vi "Nahid Final.vi"() -> ()   [LabVIEW 2019]
uses:
  <vilib>/robotics/Controls/Attitude Indicator/Attitude Indicator.xctl
  <vilib>/robotics/Controls/Compass Indicator/Compass Indicator.xctl
  <vilib>/Instr/_visa.llb/VISA Configure Serial Port (Instr).vi
panel:
  in  "byte count":u32
  in  "Speed":u32
  in  "VISA resource name":refnum<visa-resource-name>
  out "read buffer":string
  in  "Stop Button":bool
  out "Accelerometer Z":dynamicdata(graph)
  out "Accelerometer Y":dynamicdata(graph)
  out "Accelerometer X":dynamicdata(graph)
  out "Gyroscope Z":dynamicdata(graph)
  out "Gyroscope Y":dynamicdata(graph)
  out "Gyroscope X":dynamicdata(graph)
  out "Direction":dbl
  out "Thermometer":dbl(slide) scale=-2.0..100.0
  out "Low":bool
  out "Moderate":bool
  out "High":bool
  out "Temperature":dbl
  out "Humidity":dbl(slide) scale=0.0..100.0
  out "Yaw":dbl
  out "Pitch":dbl
  out "Roll":dbl
  out "Acc  Z":dbl
  out "Acc  Y":dbl
  out "Acc  X":dbl
  out "Gyro Z":dbl
  out "Gyro Y":dbl
  out "Gyro X":dbl
  out "Pressure":dbl(knob) scale=0.0..100.0
  out "Pressure":dbl
  out "Humidity":dbl
  out "Compass Indicator":dbl(xcontrol)
  out "Attitude Indicator":cluster{"Roll":dbl, "Pitch":dbl}(xcontrol)
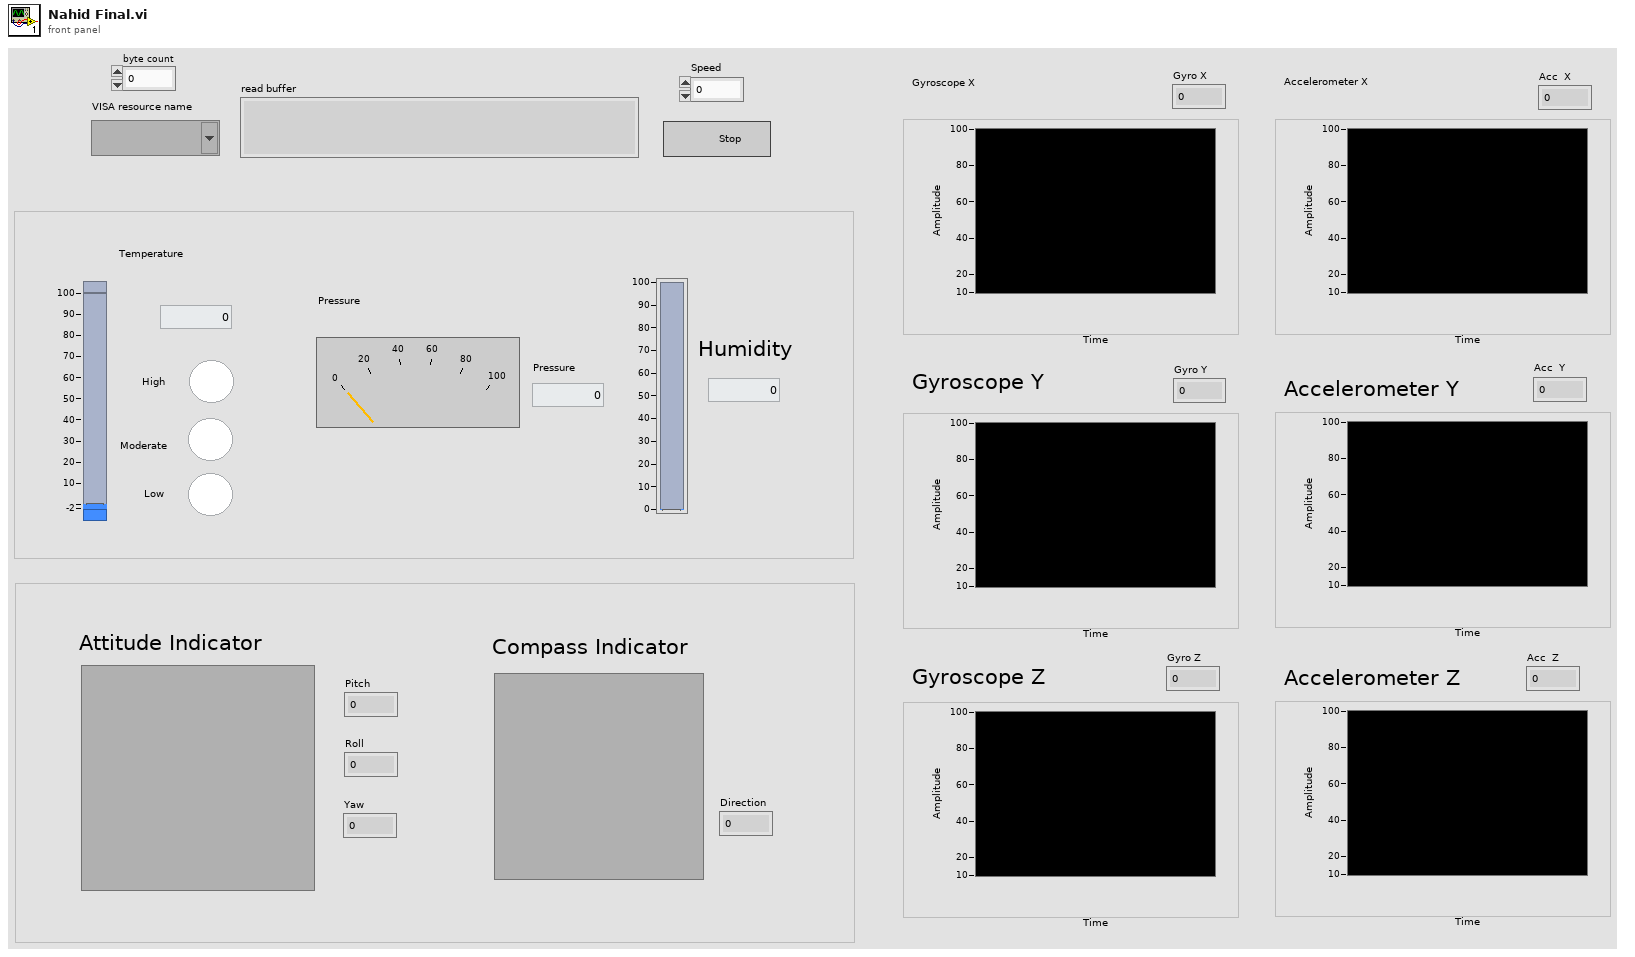
[diagram p1: front panel]
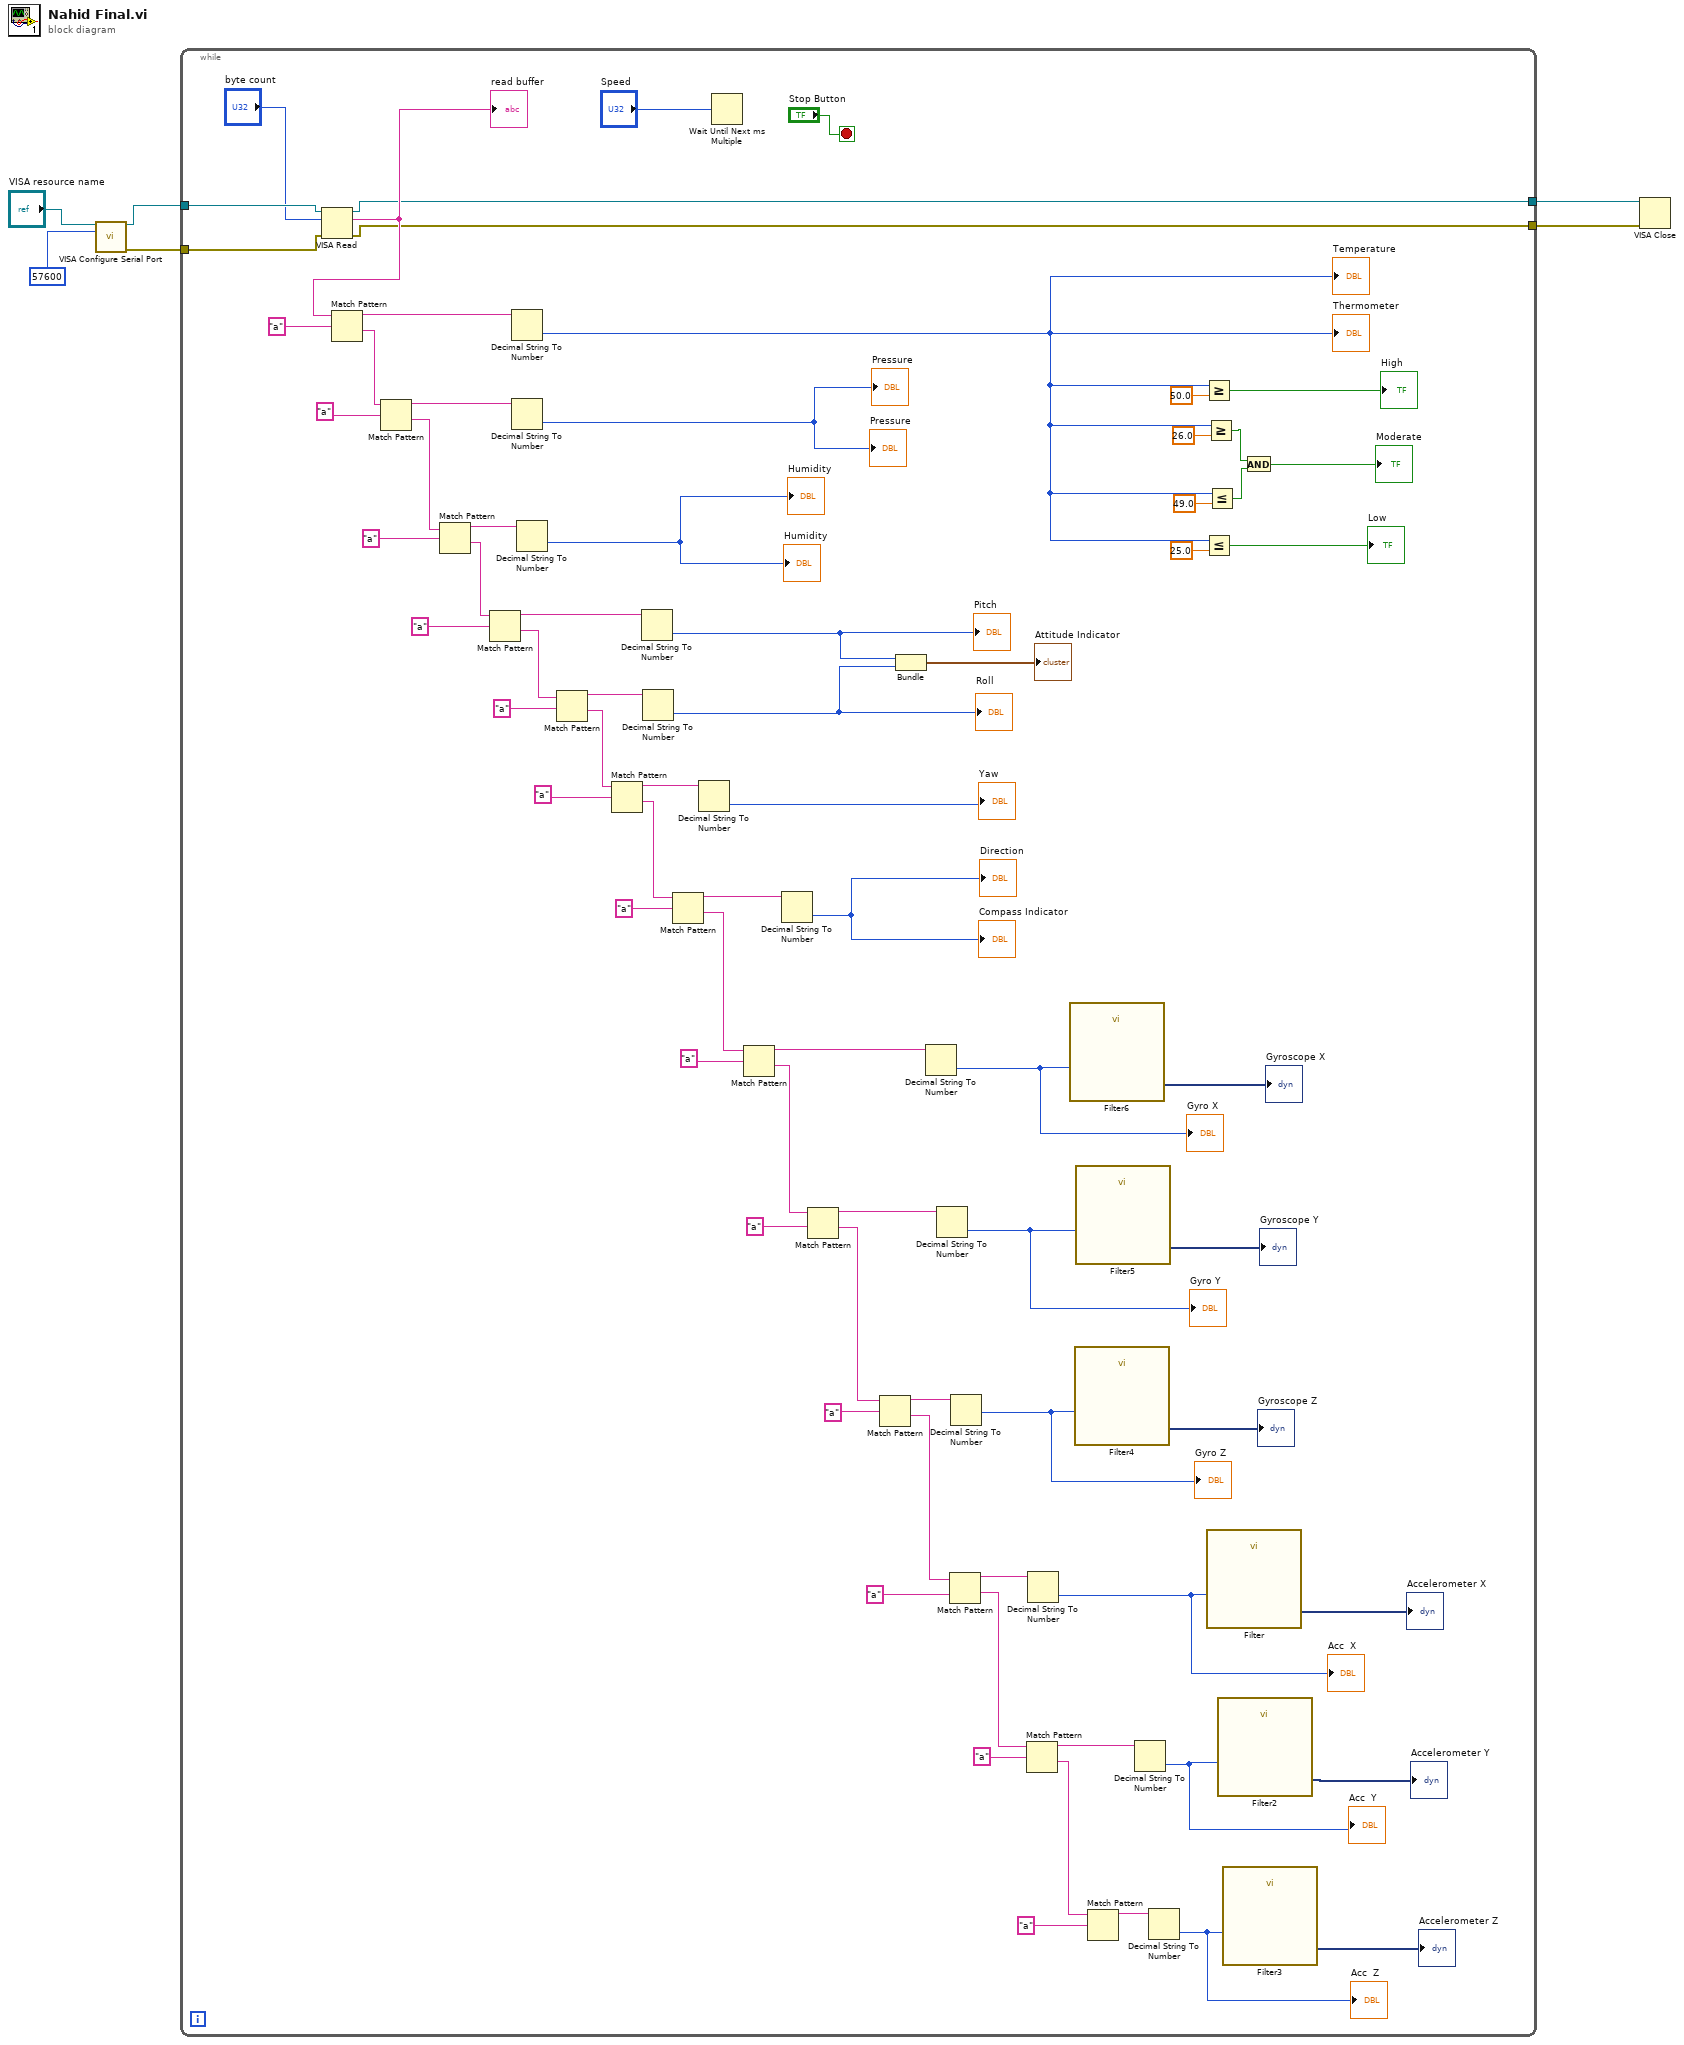
[diagram p0: block diagram]
diagram:
  n1 = call-poly "VISA Configure Serial Port"("VISA resource name"="VISA resource name", "baud rate (9600)"=u32 57600) -> ("VISA resource name out"=w4:refnum<visa-resource-name>, "error out"=w3:errorcluster)  [unwired: 12 in]
  n2 = while {
    tunnel: w4 -> [w63]
    tunnel: w3 -> [w62]
    tunnel: [w61] -> w2
    tunnel: [w60] -> w1
    stop <- "Stop Button" stop-if-true
    n3 = VISA Read(VISA resource name=w63, byte count="byte count", error in (no error)=w62) -> (VISA resource name out=w61:refnum<visa-resource-name>, read buffer=w68:string, error out=w60:errorcluster)  [unwired: 1 out]
    "read buffer" <- w68
    n4 = Match Pattern(string=w68, regular expression="a") -> (before substring=w65:string, after substring=w18:string)  [unwired: 1 in, 2 out]
    n5 = Match Pattern(string=w18, regular expression="a") -> (before substring=w70:string, after substring=w66:string)  [unwired: 1 in, 2 out]
    n6 = Match Pattern(string=w66, regular expression="a") -> (before substring=w64:string, after substring=w67:string)  [unwired: 1 in, 2 out]
    n7 = Match Pattern(string=w67, regular expression="a") -> (before substring=w58:string, after substring=w53:string)  [unwired: 1 in, 2 out]
    n8 = Decimal String To Number(string=w65) -> (number=w59:i32)  [unwired: 2 in, 1 out]
    "Temperature" <- w59
    "Thermometer" <- w59
    n9 = Decimal String To Number(string=w70) -> (number=→"Pressure" →"Pressure":i32)  [unwired: 2 in, 1 out]
    n10 = Decimal String To Number(string=w64) -> (number=→"Humidity" →"Humidity":i32)  [unwired: 2 in, 1 out]
    n11 = Match Pattern(string=w53, regular expression="a") -> (before substring=w56:string, after substring=w57:string)  [unwired: 1 in, 2 out]
    n12 = Match Pattern(string=w57, regular expression="a") -> (before substring=w54:string, after substring=w38:string)  [unwired: 1 in, 2 out]
    n13 = Decimal String To Number(string=w58) -> (number=w8:i32)  [unwired: 2 in, 1 out]
    "Pitch" <- w8
    n14 = Decimal String To Number(string=w56) -> (number=w52:i32)  [unwired: 2 in, 1 out]
    "Roll" <- w52
    n15 = Match Pattern(string=w38, regular expression="a") -> (before substring=w46:string, after substring=w49:string)  [unwired: 1 in, 2 out]
    n16 = Decimal String To Number(string=w54) -> (number=→"Yaw":i32)  [unwired: 2 in, 1 out]
    n17 = Wait Until Next ms Multiple(millisecond multiple="Speed") -> ()  [unwired: 1 out]
    n18 = Match Pattern(string=w49, regular expression="a") -> (before substring=w50:string, after substring=w47:string)  [unwired: 1 in, 2 out]
    n19 = Decimal String To Number(string=w46) -> (number=→"Compass Indicator" →"Direction":i32)  [unwired: 2 in, 1 out]
    n20 = Match Pattern(string=w47, regular expression="a") -> (before substring=w45:string, after substring=w9:string)  [unwired: 1 in, 2 out]
    n21 = Match Pattern(string=w9, regular expression="a") -> (before substring=w44:string, after substring=w40:string)  [unwired: 1 in, 2 out]
    n22 = Bundle(w8, w52) -> (→"Attitude Indicator":cluster{i32, i32})  [unwired: 1 in]
    n23 = Decimal String To Number(string=w50) -> (number=w22:i32)  [unwired: 2 in, 1 out]
    "Gyro X" <- w22
    n24 = Decimal String To Number(string=w45) -> (number=w17:i32)  [unwired: 2 in, 1 out]
    "Gyro Y" <- w17
    n25 = Match Pattern(string=w40, regular expression="a") -> (before substring=w42:string, after substring=w43:string)  [unwired: 1 in, 2 out]
    n26 = Decimal String To Number(string=w44) -> (number=w15:i32)  [unwired: 2 in, 1 out]
    "Gyro Z" <- w15
    n27 = Match Pattern(string=w43, regular expression="a") -> (before substring=w41:string, after substring=w36:string)  [unwired: 1 in, 2 out]
    n28 = Decimal String To Number(string=w42) -> (number=w13:i32)  [unwired: 2 in, 1 out]
    "Acc  X" <- w13
    n29 = call "Filter6"("Signal"=w22) -> ("Filtered Signal"=→"Gyroscope X":dynamicdata)  [unwired: 9 in, 1 out]
    n30 = call "Filter4"("Signal"=w15) -> ("Filtered Signal"=→"Gyroscope Z":dynamicdata)  [unwired: 9 in, 1 out]
    n31 = call "Filter5"("Signal"=w17) -> ("Filtered Signal"=→"Gyroscope Y":dynamicdata)  [unwired: 9 in, 1 out]
    n32 = Match Pattern(string=w36, regular expression="a") -> (before substring=w34:string)  [unwired: 1 in, 3 out]
    n33 = Decimal String To Number(string=w41) -> (number=w23:i32)  [unwired: 2 in, 1 out]
    "Acc  Y" <- w23
    n34 = Decimal String To Number(string=w34) -> (number=w10:i32)  [unwired: 2 in, 1 out]
    "Acc  Z" <- w10
    n35 = Greater Or Equal?(x=w59, y=50.0) -> (x >= y?=→"High":bool)
    n36 = Less Or Equal?(x=w59, y=25.0) -> (x <= y?=→"Low":bool)
    n37 = Greater Or Equal?(x=w59, y=26.0) -> (x >= y?=w76:bool)
    n38 = Less Or Equal?(x=w59, y=49.0) -> (x <= y?=w77:bool)
    n39 = call "Filter"("Signal"=w13) -> ("Filtered Signal"=→"Accelerometer X":dynamicdata)  [unwired: 9 in, 1 out]
    n40 = call "Filter2"("Signal"=w23) -> ("Filtered Signal"=→"Accelerometer Y":dynamicdata)  [unwired: 9 in, 1 out]
    n41 = call "Filter3"("Signal"=w10) -> ("Filtered Signal"=→"Accelerometer Z":dynamicdata)  [unwired: 9 in, 1 out]
    n42 = And(x=w76, y=w77) -> (x .and. y?=→"Moderate":bool)
  }
  n43 = VISA Close(VISA resource name=w2, error in (no error)=w1) -> ()  [unwired: 1 out]
